vi "Begin.vi"(8 "error in":errorcluster) -> (0 "error out":errorcluster)   [LabVIEW 2017]
doc: "Called before other user functions, this VI is expected to open initial I/O refnums, load in file data, and do all program initialization. Notice that the <B>error out</B> terminal is simply used for data flow. Wiring it to other structures or subVIs ensures that this VI runs first."
uses:
  <vilib>/Rock Robotics/WPI/Joystick/WPI_JoystickDeviceEnum.ctl
  <vilib>/Rock Robotics/SystemInterfaces/AI/FPGA_AIChannel.ctl
  <vilib>/Rock Robotics/SystemInterfaces/spilib/spi_bus.ctl
  <vilib>/Rock Robotics/SystemInterfaces/DIO/FPGA_DIOChannel.ctl
  SwerveRewrite/SwerveGlobals.vi
  navx-mxp/labview/navX Library v2/IO/Open/Z900_navX_Open_SPI.vi
  <vilib>/Rock Robotics/WPI/Counter/WPI_CounterDigitalInputToDigitalSource.vi
  navx-mxp/labview/navX Library v2/navX Library v2.lvlib
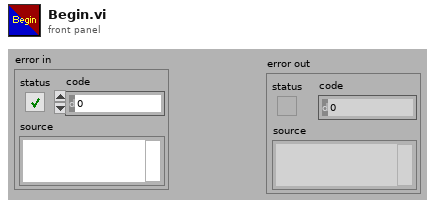
[diagram p1: front panel]
types:
  T1 = typedef "WPI_JoystickDeviceEnum.ctl" = enum16{"USB 0", "USB 1", "USB 2", "USB 3", "USB 4", "USB 5"}
  T2 = typedef "FPGA_AIChannel.ctl" = enum8{"AI 0", "AI 1", "AI 2", "AI 3", "AI MXP 0", "AI MXP 1", "AI MXP 2", "AI MXP 3", "Invalid"}
  T3 = typedef "spi_bus.ctl" = enum16{"SPI On-Board, CS0", "SPI On-Board, CS1", "SPI On-Board, CS2", "SPI On-Board, CS3", "SPI MXP", "Invalid"}
  T4 = typedef "WPI_JoystickDevRef.ctl" = cluster{"Device":T1}
  T5 = typedef "WPI_MotorControlDeviceRef.ctl" = cluster{"DeviceStatus":errorcluster, "Type":T6, "PWM":cluster{"PWM Channel":T7, "DeadBand":T8}, "CAN":cluster{"Device Number":u8, "SetOutput VI Ref":variant, "GetOutput VI Ref":variant, "Enable VI Ref":variant, "Disable VI Ref":variant, "Data":variant}, "Invert":bool, "DIO PWM":cluster{"PWM \"Enable\" Channel":T7, "DIOChannel":T9, "PWM Rate":dbl}}
  T6 = typedef "WPI_MotorControlType.ctl" = enum16{"PWM", "CAN", "DIO PWM"}
  T7 = typedef "FPGA_DIOPWMChannel.ctl" = enum8{"PWM 0", "PWM 1", "PWM 2", "PWM 3", "PWM 4", "PWM 5", "PWM 6", "PWM 7", "PWM 8", "PWM 9", "PWM MXP 0", "PWM MXP 1", "PWM MXP 2", "PWM MXP 3", "PWM MXP 4", "PWM MXP 5", "PWM MXP 6", "PWM MXP 7", "PWM MXP 8", "PWM MXP 9", "Invalid"}
  T8 = typedef "WPI_PWMDeadband.ctl" = cluster{"Name":string, "maxPositivePwm":i32, "minPositivePwm":i32, "centerPwm":i32, "maxNegativePwm":i32, "minNegativePwm":i32, "angularRange":u16}
  T9 = typedef "FPGA_DIOChannel.ctl" = enum8{"DIO 0", "DIO 1", "DIO 2", "DIO 3", "DIO 4", "DIO 5", "DIO 6", "DIO 7", "DIO 8", "DIO 9", "DIO MXP 0", "DIO MXP 1", "DIO MXP 2", "DIO MXP 3", "DIO MXP 4", "DIO MXP 5", "DIO MXP 6", "DIO MXP 7", "DIO MXP 8", "DIO MXP 9", "DIO MXP 10", "DIO MXP 11", "DIO MXP 12", "DIO MXP 13", "DIO MXP 14", "DIO MXP 15", "SPI Port CS1", "SPI Port CS2", "SPI Port CS3", "SPI Port MISO", "SPI Port MOSI", "Invalid"}
  T10 = typedef "WPI_AnalogChannelDevRef.ctl" = cluster{"DevStatus":errorcluster, "Analog Channel":T2}
  T11 = typedef "WPI_DigitalInputDevRef.ctl" = cluster{"DevStatus":errorcluster, "DIO Channel":T9}
  T12 = typedef "navX Library v2.lvlib/Z900_navX_DeviceTypeDef.ctl" = cluster{"Interface":cluster{"Protocol":T13, "Update Rate (4Hz-100Hz)":u8, "navX Open TypeDef":variant}, "Notify Packet":refnum<notifier>, "Loop VI Refnum":refnum<vi>, "Ready to Close Occurrence Refnum":refnum<k4>}
  T13 = typedef "navX Library v2.lvlib/Z900_navX_ProtocolTypeDef.ctl" = enum16{"SERIAL", "I2C", "SPI"}
  T14 = typedef "FPGA_CounterEncoderSourceConvertionLVSourceType.ctl" = cluster{"DevStatus":errorcluster, "AnalogTriggerMode?":bool, "DigitalMode":cluster{"DIO Channel":T15}, "AnalogTriggerMode":cluster{"AnalogTriggerIndex":T16, "OutputType":T17}}
  T15 = typedef "FPGA_DIODigitalSourceChannel.ctl" = enum8{"DIO 0", "DIO 1", "DIO 2", "DIO 3", "DIO 4", "DIO 5", "DIO 6", "DIO 7", "DIO 8", "DIO 9", "DIO MXP 0", "DIO MXP 1", "DIO MXP 2", "DIO MXP 3", "DIO MXP 4", "DIO MXP 5", "DIO MXP 6", "DIO MXP 7", "DIO MXP 8", "DIO MXP 9", "DIO MXP 10", "DIO MXP 11", "DIO MXP 12", "DIO MXP 13", "DIO MXP 14", "DIO MXP 15", "Disabled"}
  T16 = typedef "FPGA_AnalogTriggerIndex.ctl" = enum8{"Trig 0", "Trig 1", "Trig 2", "Trig 3", "Trig 4", "Trig 5", "Trig 6", "Trig 7", "Invalid"}
  T17 = typedef "FPGA_AnalogTriggerOutType.ctl" = enum16{"InWindow", "TriggerState", "Rising", "Falling"}
  T18 = typedef "WPI_EncoderDevRef.ctl" = cluster{"DevStatus":errorcluster, "EncoderIndex":T19, "CounterIndex":T20, "DistancePerCount":dbl, "Decoding Type":T21}
  T19 = typedef "FPGA_EncoderIdx.ctl" = enum8{"Enc 0", "Enc 1", "Enc 2", "Enc 3", "Enc 4", "Enc 5", "Enc 6", "Enc 7", "Invalid"}
  T20 = typedef "FPGA_CounterCtrSystemIndex.ctl" = enum8{"Ctr 0", "Ctr 1", "Ctr 2", "Ctr 3", "Ctr 4", "Ctr 5", "Ctr 6", "Ctr 7", "Invalid"}
  T21 = typedef "WPI_EncoderType.ctl" = enum16{"1x", "2x", "4x"}
  T22 = cluster{"Yaw":dbl, "Roll":dbl, "Pitch":dbl, "Heading":dbl, "Fused Heading":dbl}
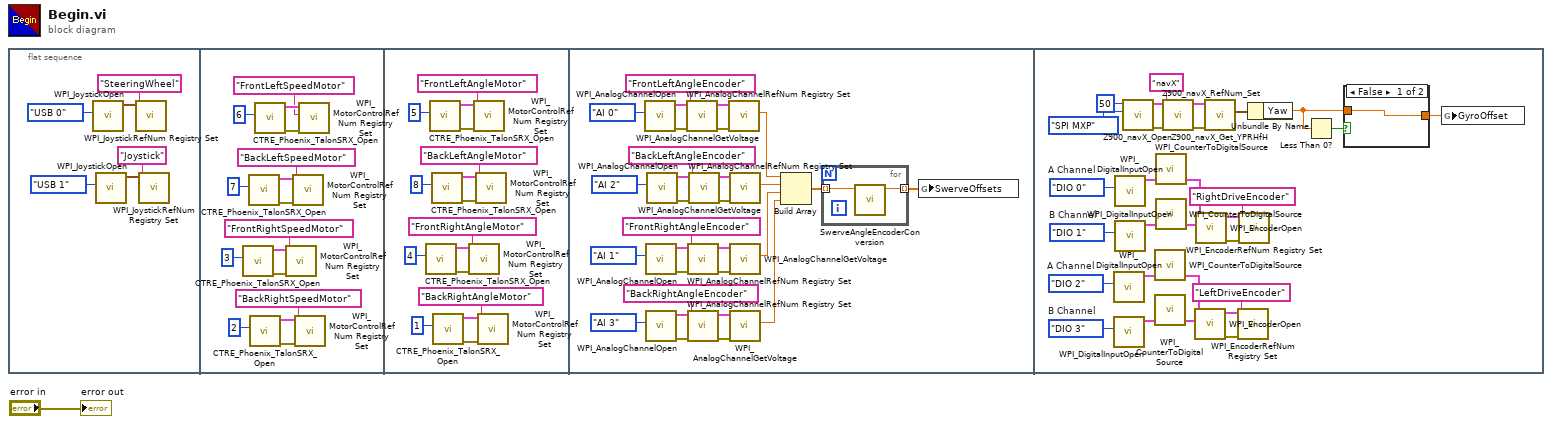
[diagram p0: block diagram]
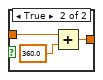
[diagram p2: hidden frame]
diagram:
  n1 = flat-sequence {
    frame #0 {
      n2 = call <vilib>:"WPI_JoystickOpen.vi"("JoystickDevice"=WPI_JoystickDeviceEnum."USB 0") -> ("JoystickDevRef"=w7:T4)  [unwired: 10 in]
      n3 = call <vilib>:"WPI_JoystickOpen.vi"("JoystickDevice"=WPI_JoystickDeviceEnum."USB 1") -> ("JoystickDevRef"=w4:T4)  [unwired: 10 in]
      n4 = call <vilib>:"WPI_JoystickRefNum Registry Set.vi"("refnum name"="SteeringWheel", "JoystickDevRef"=w7) -> ()  [unwired: 8 in, 2 out]
      n5 = call <vilib>:"WPI_JoystickRefNum Registry Set.vi"("refnum name"="Joystick", "JoystickDevRef"=w4) -> ()  [unwired: 8 in, 2 out]
    }
    frame #1 {
      n6 = call <vilib>:"CTRE_Phoenix_TalonSRX_Open.vi"("Device Number"=u8 3) -> ("error out"=w19:errorcluster, "CAN Talon SRX Ref"=w18:T5)  [unwired: 9 in]
      n7 = call <vilib>:"CTRE_Phoenix_TalonSRX_Open.vi"("Device Number"=u8 7) -> ("error out"=w21:errorcluster, "CAN Talon SRX Ref"=w20:T5)  [unwired: 9 in]
      n8 = call <vilib>:"CTRE_Phoenix_TalonSRX_Open.vi"("Device Number"=u8 2) -> ("error out"=w23:errorcluster, "CAN Talon SRX Ref"=w22:T5)  [unwired: 9 in]
      n9 = call <vilib>:"CTRE_Phoenix_TalonSRX_Open.vi"("Device Number"=u8 6) -> ("error out"=w11:errorcluster, "CAN Talon SRX Ref"=w10:T5)  [unwired: 9 in]
      n10 = call <vilib>:"WPI_MotorControlRefNum Registry Set.vi"("error in (no error)"=w19, "refnum name"="FrontRightSpeedMotor", "MotorControlDevRef"=w18) -> ()  [unwired: 7 in, 2 out]
      n11 = call <vilib>:"WPI_MotorControlRefNum Registry Set.vi"("error in (no error)"=w21, "refnum name"="BackLeftSpeedMotor", "MotorControlDevRef"=w20) -> ()  [unwired: 7 in, 2 out]
      n12 = call <vilib>:"WPI_MotorControlRefNum Registry Set.vi"("error in (no error)"=w23, "refnum name"="BackRightSpeedMotor", "MotorControlDevRef"=w22) -> ()  [unwired: 7 in, 2 out]
      n13 = call <vilib>:"WPI_MotorControlRefNum Registry Set.vi"("error in (no error)"=w11, "refnum name"="FrontLeftSpeedMotor", "MotorControlDevRef"=w10) -> ()  [unwired: 7 in, 2 out]
    }
    frame #2 {
      n14 = call <vilib>:"CTRE_Phoenix_TalonSRX_Open.vi"("Device Number"=u8 4) -> ("error out"=w34:errorcluster, "CAN Talon SRX Ref"=w35:T5)  [unwired: 9 in]
      n15 = call <vilib>:"CTRE_Phoenix_TalonSRX_Open.vi"("Device Number"=u8 5) -> ("error out"=w29:errorcluster, "CAN Talon SRX Ref"=w30:T5)  [unwired: 9 in]
      n16 = call <vilib>:"CTRE_Phoenix_TalonSRX_Open.vi"("Device Number"=u8 8) -> ("error out"=w31:errorcluster, "CAN Talon SRX Ref"=w32:T5)  [unwired: 9 in]
      n17 = call <vilib>:"CTRE_Phoenix_TalonSRX_Open.vi"("Device Number"=u8 1) -> ("error out"=w27:errorcluster, "CAN Talon SRX Ref"=w28:T5)  [unwired: 9 in]
      n18 = call <vilib>:"WPI_MotorControlRefNum Registry Set.vi"("error in (no error)"=w34, "refnum name"="FrontRightAngleMotor", "MotorControlDevRef"=w35) -> ()  [unwired: 7 in, 2 out]
      n19 = call <vilib>:"WPI_MotorControlRefNum Registry Set.vi"("error in (no error)"=w29, "refnum name"="FrontLeftAngleMotor", "MotorControlDevRef"=w30) -> ()  [unwired: 7 in, 2 out]
      n20 = call <vilib>:"WPI_MotorControlRefNum Registry Set.vi"("error in (no error)"=w31, "refnum name"="BackLeftAngleMotor", "MotorControlDevRef"=w32) -> ()  [unwired: 7 in, 2 out]
      n21 = call <vilib>:"WPI_MotorControlRefNum Registry Set.vi"("error in (no error)"=w27, "refnum name"="BackRightAngleMotor", "MotorControlDevRef"=w28) -> ()  [unwired: 7 in, 2 out]
    }
    frame #3 {
      n22 = call <vilib>:"WPI_AnalogChannelOpen.vi"("Analog Channel"=FPGA_AIChannel."AI 0") -> ("error out"=w68:errorcluster, "AIDeviceRef"=w69:T10)  [unwired: 9 in]
      n23 = call <vilib>:"WPI_AnalogChannelOpen.vi"("Analog Channel"=FPGA_AIChannel."AI 1") -> ("error out"=w60:errorcluster, "AIDeviceRef"=w61:T10)  [unwired: 9 in]
      n24 = call <vilib>:"WPI_AnalogChannelOpen.vi"("Analog Channel"=FPGA_AIChannel."AI 3") -> ("error out"=w56:errorcluster, "AIDeviceRef"=w57:T10)  [unwired: 9 in]
      n25 = call <vilib>:"WPI_AnalogChannelOpen.vi"("Analog Channel"=FPGA_AIChannel."AI 2") -> ("error out"=w64:errorcluster, "AIDeviceRef"=w65:T10)  [unwired: 9 in]
      n26 = call <vilib>:"WPI_AnalogChannelRefNum Registry Set.vi"("error in (no error)"=w68, "refnum name"="FrontLeftAngleEncoder", "AIDeviceRef"=w69) -> ("error out"=w52:errorcluster, "AIDeviceRef"=w53:T10)  [unwired: 7 in]
      n27 = call <vilib>:"WPI_AnalogChannelRefNum Registry Set.vi"("error in (no error)"=w60, "refnum name"="FrontRightAngleEncoder", "AIDeviceRef"=w61) -> ("error out"=w48:errorcluster, "AIDeviceRef"=w49:T10)  [unwired: 7 in]
      n28 = call <vilib>:"WPI_AnalogChannelRefNum Registry Set.vi"("error in (no error)"=w56, "refnum name"="BackRightAngleEncoder", "AIDeviceRef"=w57) -> ("error out"=w46:errorcluster, "AIDeviceRef"=w47:T10)  [unwired: 7 in]
      n29 = call <vilib>:"WPI_AnalogChannelRefNum Registry Set.vi"("error in (no error)"=w64, "refnum name"="BackLeftAngleEncoder", "AIDeviceRef"=w65) -> ("error out"=w50:errorcluster, "AIDeviceRef"=w51:T10)  [unwired: 7 in]
      n30 = call <vilib>:"WPI_AnalogChannelGetVoltage.vi"("error in (no error)"=w52, "AIDeviceRef"=w53) -> ("Voltage"=w45:dbl)  [unwired: 7 in, 2 out]
      n31 = call <vilib>:"WPI_AnalogChannelGetVoltage.vi"("error in (no error)"=w50, "AIDeviceRef"=w51) -> ("Voltage"=w44:dbl)  [unwired: 7 in, 2 out]
      n32 = call <vilib>:"WPI_AnalogChannelGetVoltage.vi"("error in (no error)"=w48, "AIDeviceRef"=w49) -> ("Voltage"=w43:dbl)  [unwired: 7 in, 2 out]
      n33 = call <vilib>:"WPI_AnalogChannelGetVoltage.vi"("error in (no error)"=w46, "AIDeviceRef"=w47) -> ("Voltage"=w42:dbl)  [unwired: 7 in, 2 out]
      n34 = Build Array(w45, w44, w43, w42) -> (w41:dbl[])
      n35 = for {
        tunnel: w41 -> [w71] mode=indexing
        tunnel: [w70] -> w40 mode=indexing
        n36 = call "SwerveAngleEncoderConversion.vi"("Voltage"=w71) -> ("Angle"=w70:dbl)  [unwired: 10 in]
      }
      n37 = global write "SwerveGlobals.vi" "SwerveOffsets"(w40) -> ()
    }
    frame #4 {
      w82 = FPGA_DIOChannel."DIO 3"  # B Channel
      w81 = FPGA_DIOChannel."DIO 2"  # A Channel
      w91 = FPGA_DIOChannel."DIO 1"  # B Channel
      w90 = FPGA_DIOChannel."DIO 0"  # A Channel
      n38 = call <vilib>:"WPI_DigitalInputOpen.vi"("DIO Channel"=w81) -> ("DigitalInputDevRef"=w85:T11)  [unwired: 1 in, 9 out]
      n39 = call <vilib>:"WPI_DigitalInputOpen.vi"("DIO Channel"=w82) -> ("DigitalInputDevRef"=w84:T11)  [unwired: 1 in, 9 out]
      n40 = call <vilib>:"WPI_DigitalInputOpen.vi"("DIO Channel"=w90) -> ("DigitalInputDevRef"=w94:T11)  [unwired: 1 in, 9 out]
      n41 = call <vilib>:"WPI_DigitalInputOpen.vi"("DIO Channel"=w91) -> ("DigitalInputDevRef"=w93:T11)  [unwired: 1 in, 9 out]
      n42 = call-poly "Z900_navX_Open.vi"("SPI Bus"=spi_bus."SPI MXP", "Update Rate (4Hz-60Hz)"=u8 50) -> ("error out"=w100:errorcluster, "navX Device"=w99:T12)  [unwired: 8 in]
      n43 = call-poly <vilib>:"WPI_CounterToDigitalSource.vi"("DigitalInputDevRef"=w85) -> ("Digital Source"=w86:T14)  [unwired: 6 out]
      n44 = call-poly <vilib>:"WPI_CounterToDigitalSource.vi"("DigitalInputDevRef"=w84) -> ("Digital Source"=w83:T14)  [unwired: 6 out]
      n45 = call-poly <vilib>:"WPI_CounterToDigitalSource.vi"("DigitalInputDevRef"=w94) -> ("Digital Source"=w95:T14)  [unwired: 6 out]
      n46 = call-poly <vilib>:"WPI_CounterToDigitalSource.vi"("DigitalInputDevRef"=w93) -> ("Digital Source"=w92:T14)  [unwired: 6 out]
      n47 = call "Z900_navX_RefNum_Set.vi"("error in (no error)"=w100, "refnum name"="navX", "navX Device"=w99) -> ("error out"=w75:errorcluster, "navX Device"=w76:T12)  [unwired: 7 in]
      n48 = call <vilib>:"WPI_EncoderOpen.vi"("BSource"=w83, "ASource"=w86) -> ("error out"=w80:errorcluster, "EncoderDevRef"=w79:T18)  [unwired: 6 in, 2 out]
      n49 = call <vilib>:"WPI_EncoderOpen.vi"("BSource"=w92, "ASource"=w95) -> ("error out"=w89:errorcluster, "EncoderDevRef"=w88:T18)  [unwired: 6 in, 2 out]
      n50 = call "Z900_navX_Get_YPRHfH.vi"("error in (no error)"=w75, "navX Device"=w76) -> ("YRPHfH"=w77:T22)  [unwired: 6 in, 3 out]
      n51 = call <vilib>:"WPI_EncoderRefNum Registry Set.vi"("error in (no error)"=w80, "refnum name"="LeftDriveEncoder", "EncoderDevRef"=w79) -> ()  [unwired: 7 in, 2 out]
      n52 = call <vilib>:"WPI_EncoderRefNum Registry Set.vi"("error in (no error)"=w89, "refnum name"="RightDriveEncoder", "EncoderDevRef"=w88) -> ()  [unwired: 7 in, 2 out]
      n53 = Unbundle By Name(w77) -> ("Yaw"=w73:dbl)
      n54 = Less Than 0?(x=w73) -> (x < 0?=w74:bool)
      n55 = case shown="False" w74 {
        tunnel: w73 -> [w101 w104]
        tunnel: [w101 w102] -> w72
        frame False {
        }
        frame True {
          n56 = Add(x=w104, y=360.0) -> (x+y=w102:dbl)
        }
      }
      n57 = global write "SwerveGlobals.vi" "GyroOffset"(w72) -> ()
    }
  }
  "error out" <- "error in"
